vi "Read Video.vi"(8 "error in (no error)":errorcluster, 11 "input cluster":T6={"Video Resolution"=enum."FREENECT_RESOLUTION_LOW", "Video Format"=enum."FREENECT_VIDEO_RGB", "Depth Format"=enum."FREENECT_DEPTH_11BIT", "Depth Resolution"=enum."FREENECT_RESOLUTION_LOW"}) -> (0 "error out":errorcluster, 1 "raw data":u32[][](array[numeric]), 3 "RGB image":picture)   [LabVIEW 2015]
uses:
  Video Resolution Control.ctl
  Video Format Control.ctl
  Depth Resolution Control.ctl
  <vilib>/picture/picture.llb/Draw True-Color Pixmap.vi
  libkinect_wrapper.dll
  <vilib>/vision/NI_Vision_Development_Module.lvlib
panel:
  out "Largest Particle Image":T1(plugin-control)
  in  "HSL Ranges":T2={"Hue Range"={"Lower value"=80, "Upper value"=255}, "Sat Range"={"Lower value"=0, "Upper value"=30}, "Luma Range"={"Lower value"=0, "Upper value"=60}}
  out "error out 4":errorcluster
  out "error out 3":errorcluster
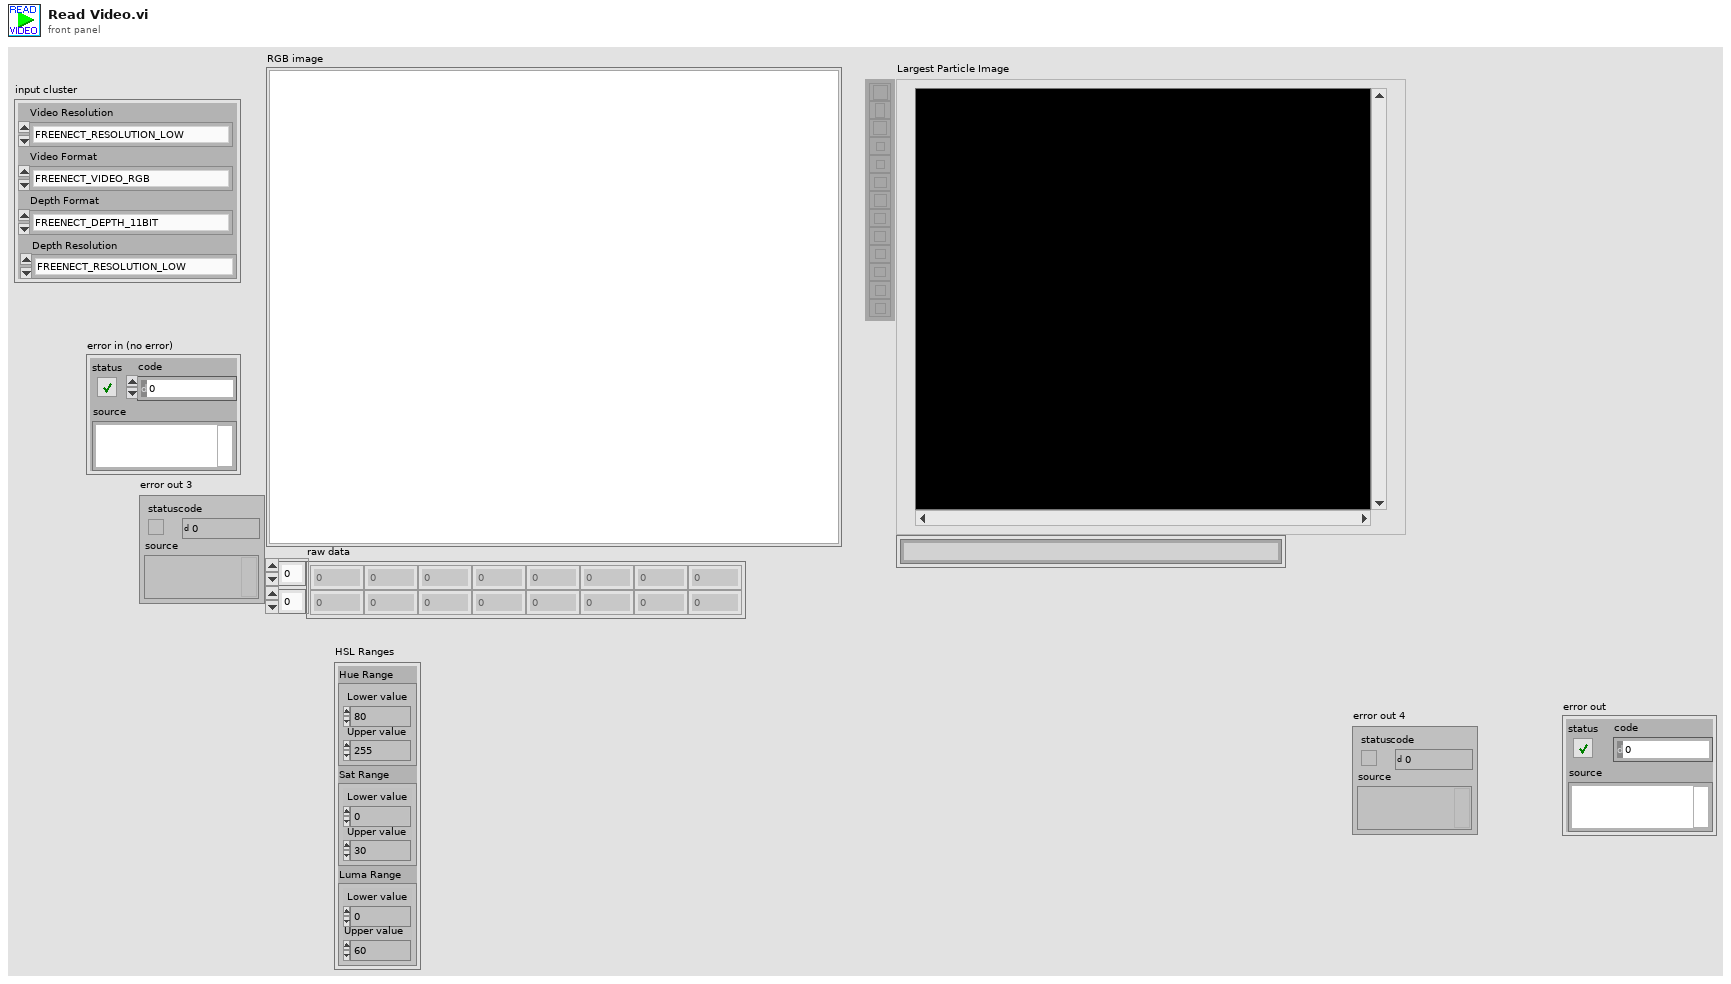
[diagram p1: front panel]
types:
  T1 = typedef "IMAQ Image.ctl" = refnum<image>
  T2 = cluster{"Hue Range":cluster{"Lower value":i32, "Upper value":i32}, "Sat Range":cluster{"Lower value":i32, "Upper value":i32}, "Luma Range":cluster{"Lower value":i32, "Upper value":i32}}
  T3 = typedef "Video Resolution Control.ctl" = enum32{"FREENECT_RESOLUTION_LOW", "FREENECT_RESOLUTION_MEDIUM", "FREENECT_RESOLUTION_HIGH"}
  T4 = typedef "Video Format Control.ctl" = enum32{"FREENECT_VIDEO_RGB", "FREENECT_VIDEO_BAYER", "FREENECT_VIDEO_IR_8BIT", "FREENECT_VIDEO_IR_10BIT", "FREENECT_VIDEO_IR_10BIT_PACKED", "FREENECT_VIDEO_YUV_RGB", "FREENECT_VIDEO_YUV_RAW"}
  T5 = typedef "Depth Resolution Control.ctl" = enum16{"FREENECT_RESOLUTION_TINY", "FREENECT_RESOLUTION_LOW", "FREENECT_RESOLUTION_MEDIUM"}
  T6 = cluster{"Video Resolution":T3, "Video Format":T4, "Depth Format":enum32{"FREENECT_DEPTH_11BIT", "FREENECT_DEPTH_10BIT", "FREENECT_DEPTH_11BIT_PACKED", "FREENECT_DEPTH_10BIT_PACKED", "FREENECT_DEPTH_REGISTERED", "FREENECT_DEPTH_MM"}, "Depth Resolution":T5}
  T7 = typedef "Image Type" = u32
  T8 = cluster{"Area":dbl, "Number of Holes":dbl, "Bounding Rect":cluster{"Left":dbl, "Top":dbl, "Right":dbl, "Bottom":dbl}, "Center of Mass":cluster{"X":dbl, "Y":dbl}, "Orientation":dbl, "Dimensions":cluster{"Width":dbl, "Height":dbl}}[]
  T9 = cluster{"Area":dbl, "Number of Holes":dbl, "Bounding Rect":cluster{"Left":dbl, "Top":dbl, "Right":dbl, "Bottom":dbl}, "Center of Mass":cluster{"X":dbl, "Y":dbl}, "Orientation":dbl, "Dimensions":cluster{"Width":dbl, "Height":dbl}}
  T10 = cluster{"Left":dbl, "Top":dbl, "Right":dbl, "Bottom":dbl}
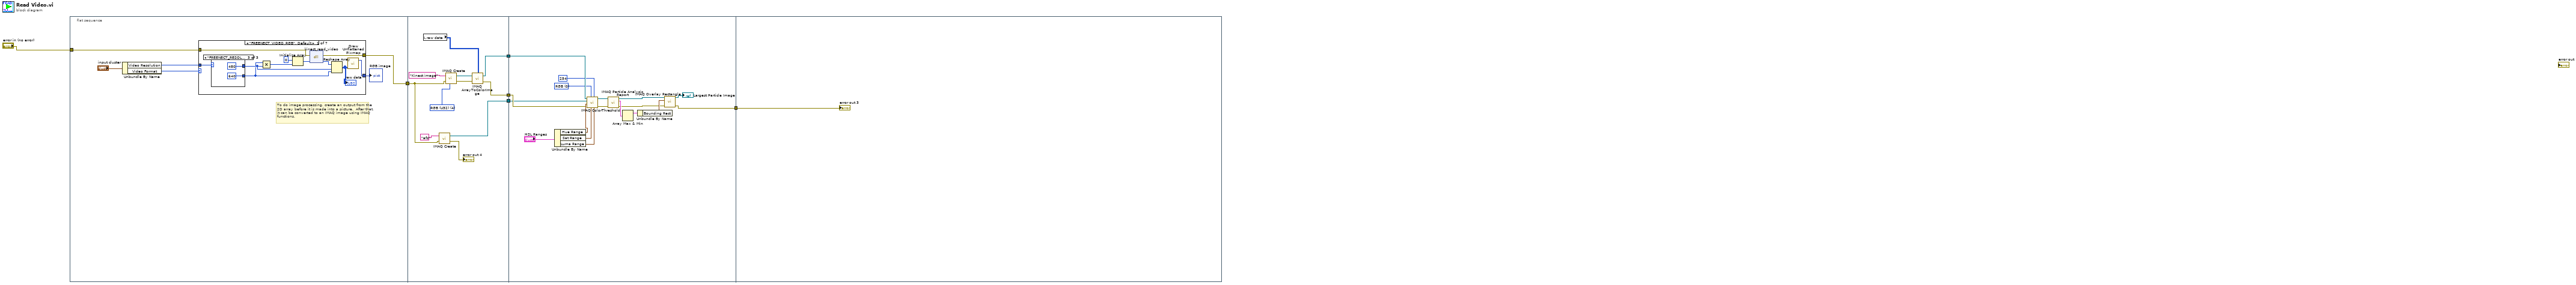
[diagram p0: block diagram]
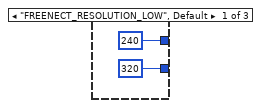
[diagram p2: hidden frame]
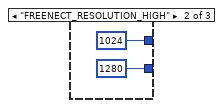
[diagram p3: hidden frame]
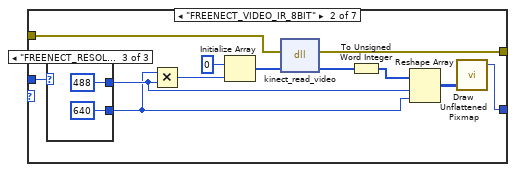
[diagram p4: hidden frame]
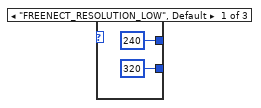
[diagram p5: hidden frame]
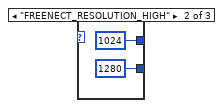
[diagram p6: hidden frame]
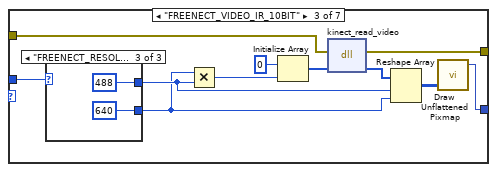
[diagram p7: hidden frame]
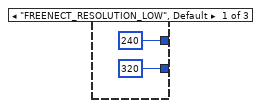
[diagram p8: hidden frame]
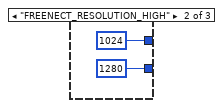
[diagram p9: hidden frame]
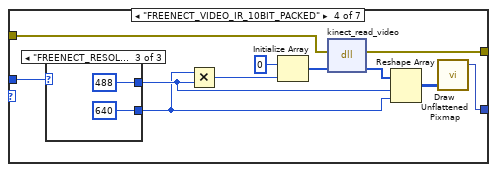
[diagram p10: hidden frame]
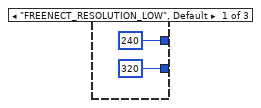
[diagram p11: hidden frame]
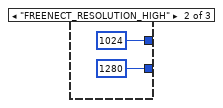
[diagram p12: hidden frame]
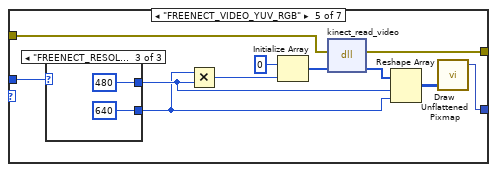
[diagram p13: hidden frame]
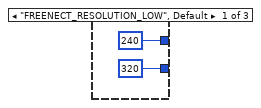
[diagram p14: hidden frame]
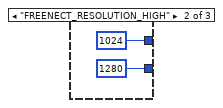
[diagram p15: hidden frame]
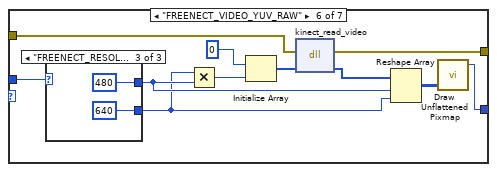
[diagram p16: hidden frame]
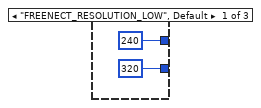
[diagram p17: hidden frame]
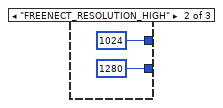
[diagram p18: hidden frame]
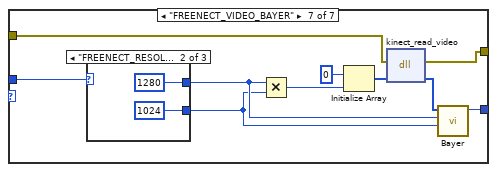
[diagram p19: hidden frame]
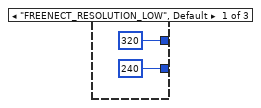
[diagram p20: hidden frame]
diagram:
  n1 = flat-sequence {
    tunnel: [w9] -> w6
    tunnel: "error in (no error)" -> [w7]
    tunnel: w6 -> [w134]
    tunnel: [w140] -> w4
    tunnel: [w136] -> w3
    tunnel: [w132] -> w2
    tunnel: w4 -> [w156]
    tunnel: w3 -> [w155]
    tunnel: w2 -> [w154]
    tunnel: [w144] -> w1
    tunnel: w1 -> [w161]
    frame #0 {
      # "To do image processing, create an output from the 2D array before it is made into a picture.  After that, it can be converted to an IMAQ image using IMAQ functions."
      n2 = Unbundle By Name("input cluster") -> ("Video Resolution"=w10:T3, "Video Format"=w11:T4)
      n3 = case shown="\"FREENECT_VIDEO_RGB\", Default" w11 {
        tunnel: w10 -> [w23 w33 w48 w67 w92 w109 w118]
        tunnel: [w19 w35 w50 w69 w86 w100 w119] -> w8
        tunnel: w7 -> [w18 w34 w49 w68 w85 w105 w121]
        tunnel: [w17 w36 w51 w70 w84 w104 w120] -> w9
        frame "FREENECT_VIDEO_RGB", Default {
          n4 = case shown="\"FREENECT_RESOLUTION_MEDIUM\"" w23 {
            tunnel: [240 1024 480] -> w16
            tunnel: [320 1280 640] -> w15
            frame "FREENECT_RESOLUTION_LOW", Default {
            }
            frame "FREENECT_RESOLUTION_HIGH" {
            }
            frame "FREENECT_RESOLUTION_MEDIUM" {
            }
          }
          n5 = Multiply(x=w15, y=w16) -> (x*y=w22:i32)
          n6 = Initialize Array(u32 0 ("U32"), w22) -> (w21:u32[])
          n7 = dll-call lib="libkinect_wrapper.*" fn="kinect_read_video"(error in=w18, "video"=w21) -> (error out=w17:errorcluster, "video"=w14:u32[])  [unwired: 3 in, 1 out]
          n8 = Reshape Array(w14, w16, w15) -> (w13:u32[][])
          "raw data" <- w13
          n9 = call-poly <vilib>:"Draw Unflattened Pixmap.vi"("data (RGB format)"=w13) -> ("new picture"=w19:picture)  [unwired: 8 in]
        }
        frame "FREENECT_VIDEO_IR_8BIT" {
          n10 = case shown="\"FREENECT_RESOLUTION_MEDIUM\"" w33 {
            tunnel: [240 1024 488] -> w38
            tunnel: [320 1280 640] -> w37
            frame "FREENECT_RESOLUTION_LOW", Default {
            }
            frame "FREENECT_RESOLUTION_HIGH" {
            }
            frame "FREENECT_RESOLUTION_MEDIUM" {
            }
          }
          n11 = Multiply(x=w37, y=w38) -> (x*y=w41:i32)
          n12 = Initialize Array(u8 0 ("U32"), w41) -> (w40:u8[])
          n13 = dll-call lib="libkinect_wrapper.*" fn="kinect_read_video"(error in=w34, "video"=w40) -> (error out=w36:errorcluster, "video"=w32:u8[])  [unwired: 3 in, 1 out]
          n14 = To Unsigned Word Integer(number=w32) -> (unsigned 16bit integer=w31:u16[])
          n15 = Reshape Array(w31, w38, w37) -> (w30:u16[][])
          n16 = call-poly <vilib>:"Draw Unflattened Pixmap.vi"("data (RGB format)"=w30) -> ("new picture"=w35:picture)  [unwired: 8 in]
        }
        frame "FREENECT_VIDEO_IR_10BIT" {
          n17 = case shown="\"FREENECT_RESOLUTION_MEDIUM\"" w48 {
            tunnel: [240 1024 488] -> w53
            tunnel: [320 1280 640] -> w52
            frame "FREENECT_RESOLUTION_LOW", Default {
            }
            frame "FREENECT_RESOLUTION_HIGH" {
            }
            frame "FREENECT_RESOLUTION_MEDIUM" {
            }
          }
          n18 = Multiply(x=w52, y=w53) -> (x*y=w58:i32)
          n19 = Initialize Array(u16 0 ("U32"), w58) -> (w57:u16[])
          n20 = dll-call lib="libkinect_wrapper.*" fn="kinect_read_video"(error in=w49, "video"=w57) -> (error out=w51:errorcluster, "video"=w55:u16[])  [unwired: 3 in, 1 out]
          n21 = Reshape Array(w55, w53, w52) -> (w54:u16[][])
          n22 = call-poly <vilib>:"Draw Unflattened Pixmap.vi"("data (RGB format)"=w54) -> ("new picture"=w50:picture)  [unwired: 8 in]
        }
        frame "FREENECT_VIDEO_IR_10BIT_PACKED" {
          n23 = case shown="\"FREENECT_RESOLUTION_MEDIUM\"" w67 {
            tunnel: [240 1024 488] -> w72
            tunnel: [320 1280 640] -> w71
            frame "FREENECT_RESOLUTION_LOW", Default {
            }
            frame "FREENECT_RESOLUTION_HIGH" {
            }
            frame "FREENECT_RESOLUTION_MEDIUM" {
            }
          }
          n24 = Multiply(x=w71, y=w72) -> (x*y=w75:i32)
          n25 = Initialize Array(u16 0 ("U32"), w75) -> (w74:u16[])
          n26 = dll-call lib="libkinect_wrapper.*" fn="kinect_read_video"(error in=w68, "video"=w74) -> (error out=w70:errorcluster, "video"=w66:u16[])  [unwired: 3 in, 1 out]
          n27 = Reshape Array(w66, w72, w71) -> (w65:u16[][])
          n28 = call-poly <vilib>:"Draw Unflattened Pixmap.vi"("data (RGB format)"=w65) -> ("new picture"=w69:picture)  [unwired: 8 in]
        }
        frame "FREENECT_VIDEO_YUV_RGB" {
          n29 = case shown="\"FREENECT_RESOLUTION_MEDIUM\"" w92 {
            tunnel: [240 1024 480] -> w83
            tunnel: [320 1280 640] -> w82
            frame "FREENECT_RESOLUTION_LOW", Default {
            }
            frame "FREENECT_RESOLUTION_HIGH" {
            }
            frame "FREENECT_RESOLUTION_MEDIUM" {
            }
          }
          n30 = Multiply(x=w82, y=w83) -> (x*y=w91:i32)
          n31 = Initialize Array(u32 0 ("U32"), w91) -> (w90:u32[])
          n32 = dll-call lib="libkinect_wrapper.*" fn="kinect_read_video"(error in=w85, "video"=w90) -> (error out=w84:errorcluster, "video"=w88:u32[])  [unwired: 3 in, 1 out]
          n33 = Reshape Array(w88, w83, w82) -> (w87:u32[][])
          n34 = call-poly <vilib>:"Draw Unflattened Pixmap.vi"("data (RGB format)"=w87) -> ("new picture"=w86:picture)  [unwired: 8 in]
        }
        frame "FREENECT_VIDEO_YUV_RAW" {
          n35 = case shown="\"FREENECT_RESOLUTION_MEDIUM\"" w109 {
            tunnel: [240 1024 480] -> w103
            tunnel: [320 1280 640] -> w102
            frame "FREENECT_RESOLUTION_LOW", Default {
            }
            frame "FREENECT_RESOLUTION_HIGH" {
            }
            frame "FREENECT_RESOLUTION_MEDIUM" {
            }
          }
          n36 = Multiply(x=w102, y=w103) -> (x*y=w108:i32)
          n37 = Initialize Array(u16 0 ("U32"), w108) -> (w107:u16[])
          n38 = dll-call lib="libkinect_wrapper.*" fn="kinect_read_video"(error in=w105, "video"=w107) -> (error out=w104:errorcluster, "video"=w101:u16[])  [unwired: 3 in, 1 out]
          n39 = Reshape Array(w101, w103, w102) -> (w99:u16[][])
          n40 = call-poly <vilib>:"Draw Unflattened Pixmap.vi"("data (RGB format)"=w99) -> ("new picture"=w100:picture)  [unwired: 8 in]
        }
        frame "FREENECT_VIDEO_BAYER" {
          n41 = case shown="\"FREENECT_RESOLUTION_HIGH\"" w118 {
            tunnel: [320 1280 640] -> w117
            tunnel: [240 1024 480] -> w116
            frame "FREENECT_RESOLUTION_LOW", Default {
            }
            frame "FREENECT_RESOLUTION_HIGH" {
            }
            frame "FREENECT_RESOLUTION_MEDIUM" {
            }
          }
          n42 = Multiply(x=w117, y=w116) -> (x*y=w125:i32)
          n43 = Initialize Array(u8 0, w125) -> (w124:u8[])
          n44 = dll-call lib="libkinect_wrapper.*" fn="kinect_read_video"(error in=w121, "video"=w124) -> (error out=w120:errorcluster, "video"=w123:u8[])  [unwired: 3 in, 1 out]
          n45 = call "Bayer.vi"("Height"=w116, "Width"=w117, "Array"=w123) -> ("new picture"=w119:picture)  [unwired: 8 in]
        }
      }
      "RGB image" <- w8
    }
    frame #1 {
      w137 = T7 4 items=["Grayscale (U8)", "Grayscale (I16)", "Grayscale (SGL)", "Complex (CSG)", "RGB (U32)", "HSL (U32)", "RGB (U64)", "Grayscale (U16)"] ("Image Type")
      n46 = local read "raw data"() -> (w138:u32[][])
      n47 = call "IMAQ Create"("Image Name"="afs", "error in (no error)"=w134) -> ("New Image"=w132:T1, "error out"=→"error out 4":errorcluster)  [unwired: 3 in]
      n48 = call "IMAQ Create"("Image Name"="Kinect image", "Image Type"=w137, "error in (no error)"=w134) -> ("New Image"=w142:T1, "error out"=w141:errorcluster)  [unwired: 2 in]
      n49 = call "IMAQ ArrayToColorImage"("Image Pixels (U32)"=w138, "Image"=w142, "error in (no error)"=w141) -> ("Image Out"=w136:T1, "error out"=w140:errorcluster)  [unwired: 2 in]
    }
    frame #2 {
      w153 = u16 0 items=["RGB", "HSL", "HSV", "HSI"] ("Color Mode")
      n50 = Unbundle By Name("HSL Ranges") -> ("Hue Range"=w159:cluster{"Lower value":i32, "Upper value":i32}, "Sat Range"=w158:cluster{"Lower value":i32, "Upper value":i32}, "Luma Range"=w157:cluster{"Lower value":i32, "Upper value":i32})
      n51 = call "IMAQ ColorThreshold"("Blue or Luma or Val or Inten Range"=w157, "Replace Value"=254, "Green or Sat Range"=w158, "Color Mode"=w153, "error in (no error)"=w156, "Red or Hue Range"=w159, "Image Dst"=w154, "Image Src"=w155) -> ("error out"=w146:errorcluster, "Image Dst Out"=w145:T1)  [unwired: 2 in]
      n52 = call "IMAQ Particle Analysis Report"("error in (no error)"=w146, "Image"=w145) -> ("error out"=w149:errorcluster, "Particle Reports (Pixels)"=w150:T8, "Image Out (duplicate)"=w148:T1)  [unwired: 4 in, 3 out]
      n53 = Array Max & Min(array=w150) -> (max value=w147:T9)  [unwired: 3 out]
      n54 = Unbundle By Name(w147) -> ("Bounding Rect"=w151:T10)
      n55 = call "IMAQ Overlay Rectangle"("error in (no error)"=w149, "Rectangle"=w151, "Image"=w148) -> ("error out"=w144:errorcluster, "Image Out"=→"Largest Particle Image":T1)  [unwired: 7 in]
    }
    frame #3 {
      "error out 3" <- w161
    }
  }
